vi "Dashboard Main.vi"() -> ()   [LabVIEW 2017]
uses:
  <vilib>/Rock Robotics/WPI/ThirdParty/Sensors/navX/_TypeDefs/FRIC_navX_DeviceNumbersTypeDef.ctl
  <vilib>/Utility/miscctls.llb/LVRowAndColumnTypeDef.ctl
  <vilib>/event_ctls.llb/eventvkey.ctl
  <vilib>/Rock Robotics/Network Tables/NT Read Numeric Array.vi
  <vilib>/Rock Robotics/Network Tables/NT Write Boolean.vi
  <vilib>/Rock Robotics/Network Tables/NT Read Raw.vi
  <vilib>/Rock Robotics/Network Tables/NT Write Variant.vi
  <vilib>/Rock Robotics/Network Tables/NT Read Boolean.vi
  <vilib>/Rock Robotics/WPI/Dashboard/WPI_DashboardLogging Global.vi
panel:
  in  "On/Off  2":bool caption="Solenoid"
  in  "On/Off  2":bool caption="Solenoid"
  in  "Camera Settings Right":T1={"Frame Rate"=30, "Compression"=30, "Size"=1, "DB Camera Config"=FALSE} {"Frame Rate" scale=1.0..30.0; "Compression" scale=100.0..-1.0; "Size" items=["640x480", "320x240", "160x120"]}
  in  "Camera Name Right":string(combo)="No Camera Selection"
  out "Camera Info":cluster{"Mbps LED":bool, "Mbps":dbl, "fps":dbl} {"fps" format="%#.1g"; "Mbps" format="%#.1g"}
  in  "Camera Settings":T1={"Frame Rate"=30, "Compression"=30, "Size"=1, "DB Camera Config"=FALSE} {"Frame Rate" scale=1.0..30.0; "Compression" scale=100.0..-1.0; "Size" items=["640x480", "320x240", "160x120"]}
  in  "TCP":refnum<k5>
  in  "Rec Mode":enum32{"Stop", "Record", "Playback"}(radio)
  out "Robot IP":string
  out "Image Message":string="Timeout in Camera Communications"
  in  "Dashboard Tab":T2(tab)
  in  "DancePad?":bool
  out "Reverse":bool
  in  "Auto Wait":dbl
  in  "Start Positions":string(combo)="Select Autonomous ..."
  out "NT Connection":bool
  out "MotorChart R":cluster{"Numeric":dbl, "Numeric":dbl}(graph)
  out "MotorChart L":cluster{"Numeric":dbl, "Numeric":dbl}(graph)
  out "MotorSliders R":cluster{"MotorSlide1":dbl, "MotorSlide2":dbl} {"MotorSlide2" scale=-1.0..1.0 scale format="%#_2e"; "MotorSlide1" scale=-1.0..1.0 scale format="%#_2e"}
  out "MotorSliders L":cluster{"MotorSlide1":dbl, "MotorSlide2":dbl} {"MotorSlide2" scale=-1.0..1.0 scale format="%#_2e"; "MotorSlide1" scale=-1.0..1.0 scale format="%#_2e"}
  out "Gyro":dbl(knob) scale=-180.0..180.0
  out "JS1 Z":dbl(slide) scale=-1.0..1.0 scale format="%#_2e"
  out "JS1 Graph":cluster{"X":dbl, "Y":dbl}[](graph)
  out "JS1 Buttons":T3
  out "JS2 Z":dbl(slide) scale=-1.0..1.0 scale format="%#_2e"
  out "JS2 Graph":cluster{"X":dbl, "Y":dbl}[](graph)
  out "JS2 Buttons":T3
  out "Mode":T4(ring)=enum."Auto Disabled"
  in  "Auton Goalos":string(combo)="Select Autonomous ..."
  out "Slow":bool
  out "Linear Acceleration":T5
  in  "Zero":bool
  out "Camera Image Right":T6(plugin-control)
  in  "DB/String 9":string
  in  "DB/String 8":string
  in  "DB/String 7":string
  in  "DB/String 6":string
  in  "DB/String 5":string
  in  "DB/String 4":string
  in  "DB/String 3":string
  in  "DB/String 2":string
  in  "DB/String 1":string
  in  "DB/String 0":string
  in  "DB/Slider 0":dbl(slide) scale=0.0..5.0
  in  "DB/Slider 1":dbl(slide) scale=0.0..5.0
  in  "DB/Slider 2":dbl(slide) scale=0.0..5.0
  in  "DB/Slider 3":dbl(slide) scale=0.0..5.0
  out "DB/LED 3":bool
  out "DB/LED 2":bool
  out "DB/LED 1":bool
  out "DB/LED 0":bool
  in  "DB/Button 3":bool
  in  "DB/Button 2":bool
  in  "DB/Button 1":bool
  in  "DB/Button 0":bool caption="New Name"
  in  "Use Test PWMs\n(leave off for robot":bool
  in  "Auton Game Data Override for Testing":T7
  out "Vision Values":T8
  in  "Test Slider":dbl(slide) scale=0.0..100.0 scale format="%#_3g"
  in  "On/Off":bool caption="Solenoid"
  in  "Test Name":u16(ring) items=["Select the test to run..."]
  in  "Test Tree":string(tree)
  in  "Motor":cluster{"Value":dbl, "Enable":bool} {"Value" scale=-1.0..1.0 scale format="%#_3g"}
  out "Progress":T9 {"Test Progress" scale=0.0..100.0}
  in  "Rev/Fwd":cluster{"Forward":bool, "Reverse":bool}
  in  "Test Ring":u16(ring) items=["Monochrome", "Color"]
  out "Cmd Status":string
  in  "Execute Command":bool
  in  "Command Params":string[][](table)
  in  "Command Selection":i32(listbox)
  in  "CheckList":i32(listbox)
  out "Tree":string(tree)
  out "Camera Image":T6(plugin-control)
  in  "Camera Name":string(combo)="No Camera Selection"
  # "HW"
  # "HW"
  # "Joysticks"
  # "Drive Motors"
  # "Front"
  # "Right"
  # "Left"
  # "Back"
  # "This tab is a great place for autonomous settings and robot-specific values.\nPlace controls and indicators inside this tab and match name to\nDashboard Variables on robot. You can also delete this comment."
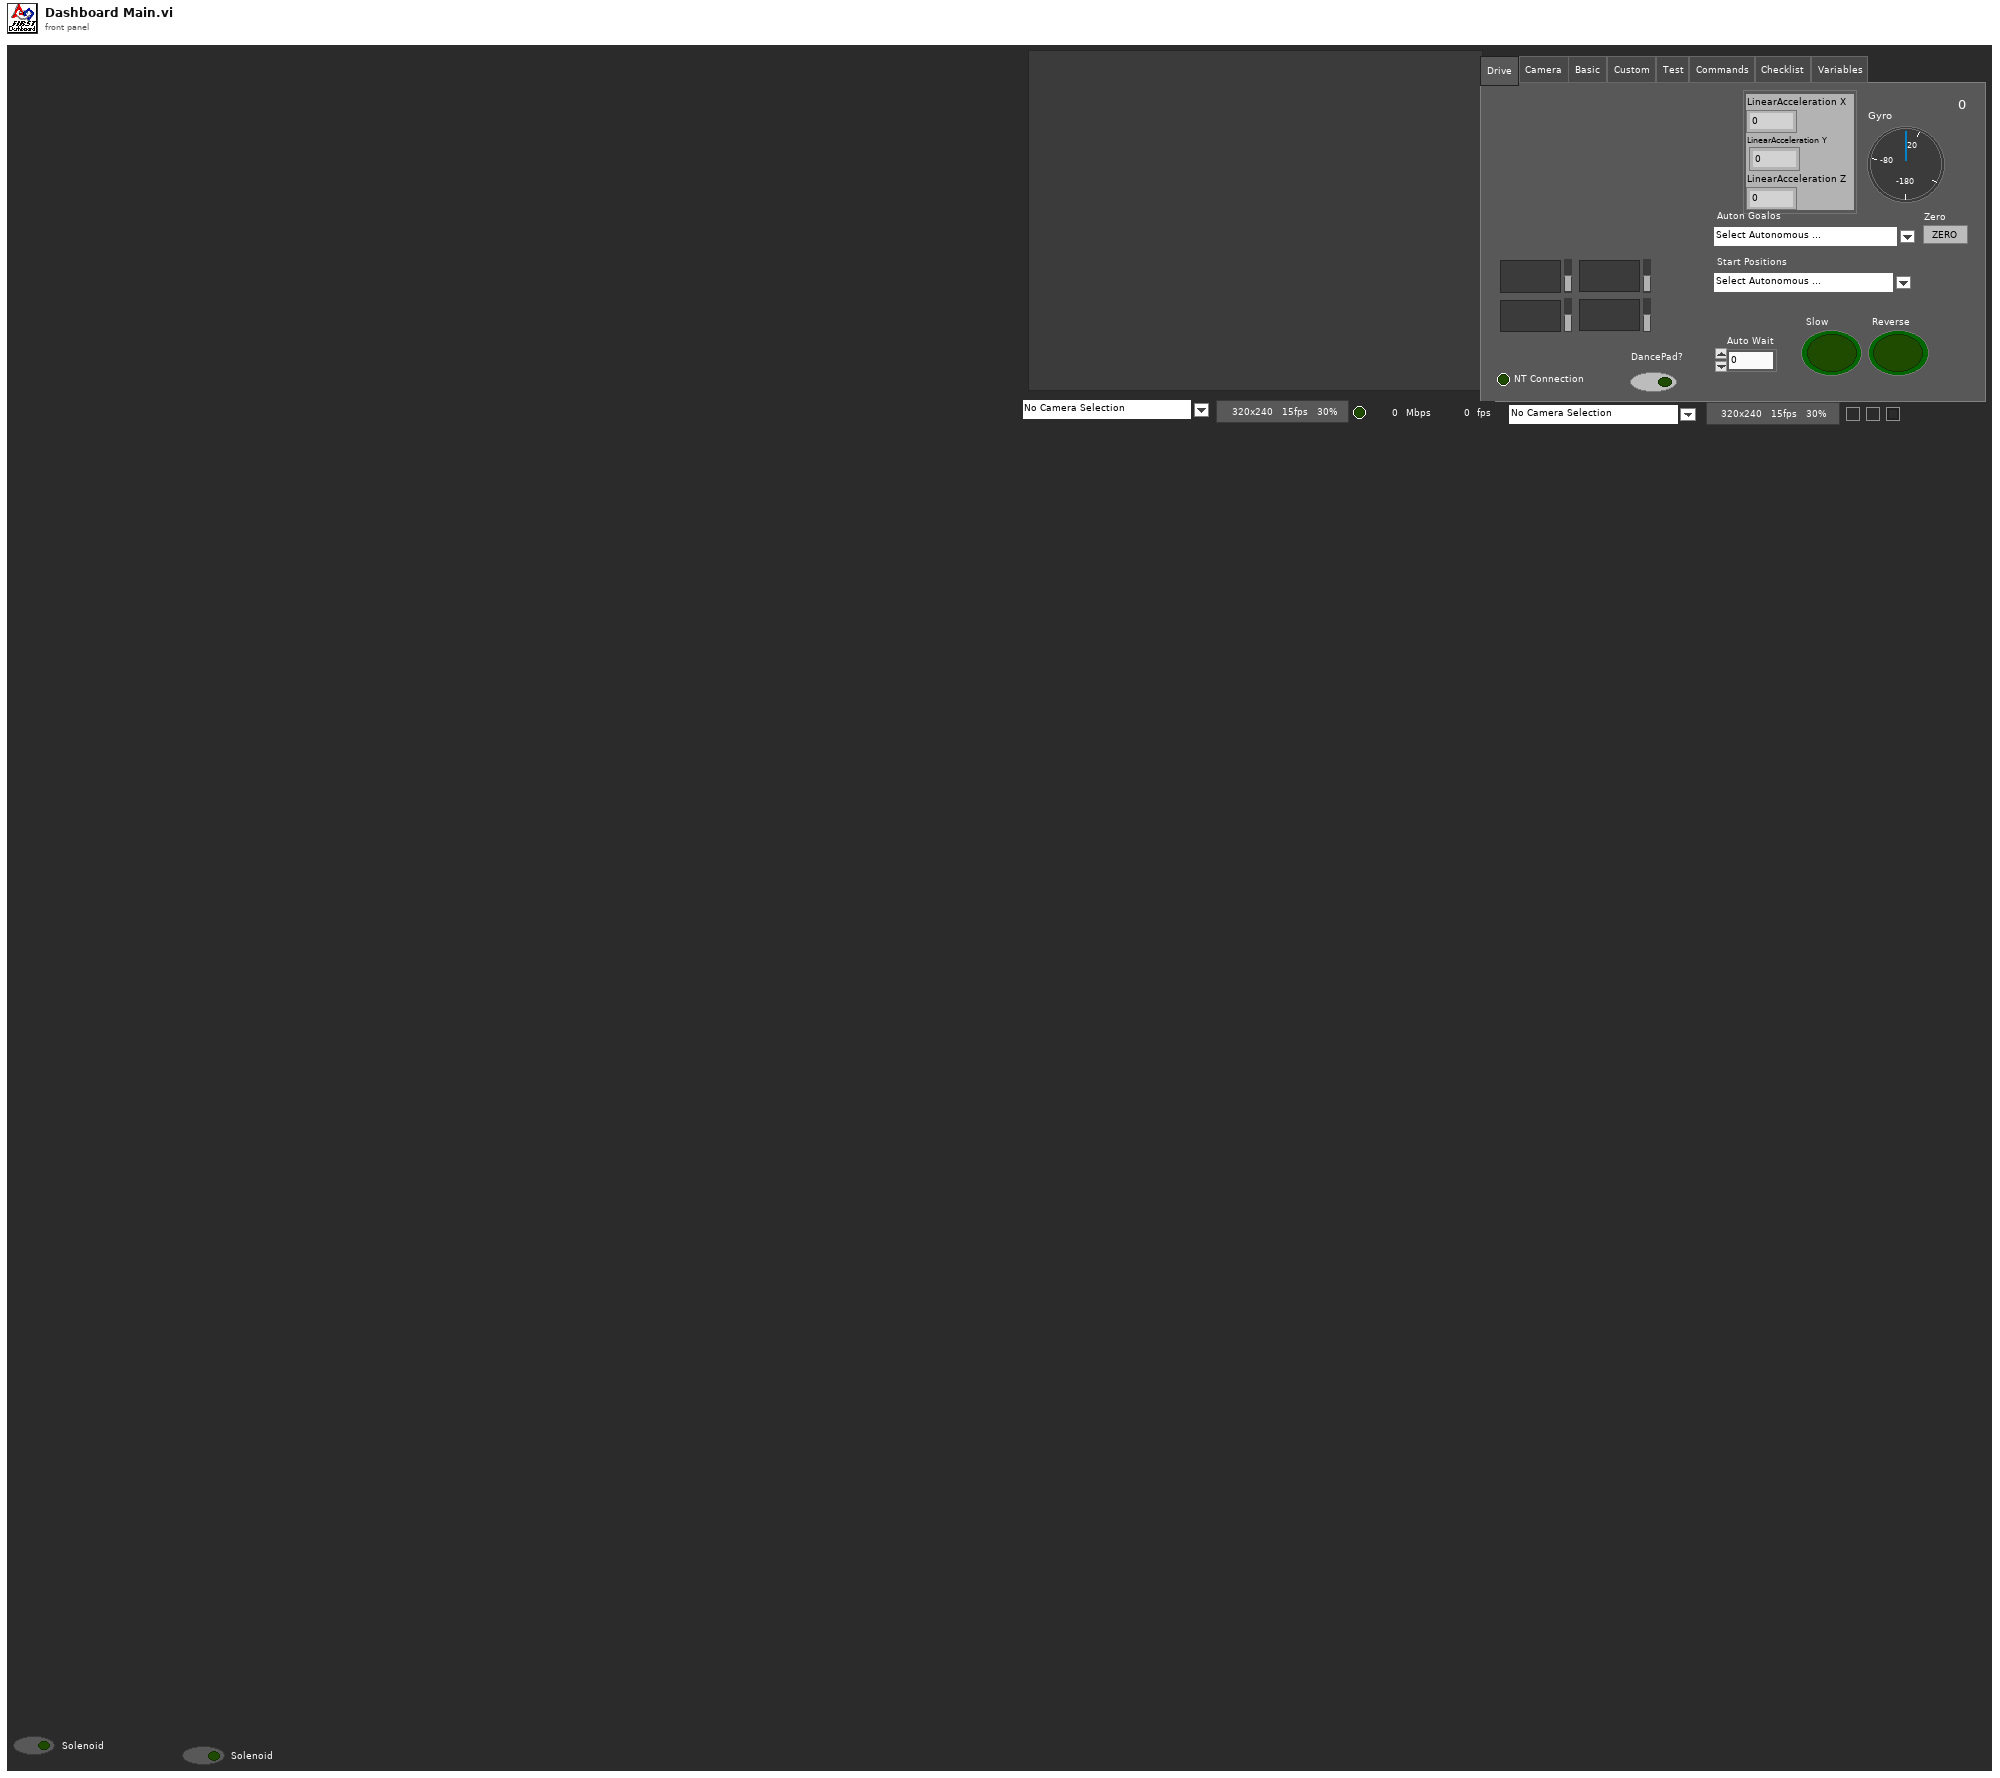
[diagram p1: front panel]
types:
  T1 = cluster{"Frame Rate":i32, "Compression":i32, "Size":u16, "DB Camera Config":bool}
  T2 = enum32{"Drive", "Camera", "Basic", "Custom", "Test", "Commands", "Checklist", "Variables"}
  T3 = cluster{bool, bool, bool, bool, bool, bool, bool, bool, bool, bool, bool, bool}
  T4 = enum8{"Tele-Op Disabled", "Tele-Op Enabled", "Auto Disabled", "Auto Enabled", "Test Disabled", "Test Enabled", "Disconnected", "No Code", "E-Stop"}
  T5 = cluster{"LinearAcceleration X":dbl, "LinearAcceleration Y":dbl, "LinearAcceleration Z":dbl}
  T6 = typedef "IMAQ Image.ctl" = refnum<image>
  T7 = cluster{"Enable":bool, "Switch Left":bool, "Scale Left":bool}
  T8 = cluster{"Center of Mass X":dbl, "Turn degrees":dbl, "Pixel Area":dbl, "Positive or Negative?":dbl}
  T9 = cluster{"Test Progress":u8, "Test Progress Text":string}
  T10 = typedef "FRIC_navX_DeviceNumbersTypeDef.ctl" = enum16{"Dev0", "Dev1", "Dev2", "Dev3"}
  T11 = cluster{"Save Path":path, "Interval (s)":dbl, "Keep":i32}
  T12 = typedef "Image Type" = u32
  T13 = cluster{"IDs":cluster{"RPC field ID":u16, "Unique ID":u16}, "String":string}
  T14 = cluster{"Error Strings":string, "Disable Counts":cluster{u16, u16}, "Rail Faults":cluster{u16, u16, u16}, "Robot IP":string, "DB Mode":u8, "Event Info":cluster{"Name":string, "Type":u8, "Number":u16, "Replay":u8}}
  T15 = cluster{"Storage":cluster{"Disk Free":u64, "RAM Block":u32, "RAM free":u32}, "CPU Utilization":cluster{"CPU % ISR":sgl, "CPU % Time Crit":sgl, "CPU % Timed Str":sgl, "CPU % High":sgl, "CPU % Above":sgl, "CPU % Normal":sgl, "CPU % Low":sgl}, "CAN":cluster{"% Bus Utilization":sgl, "Bus Off Cnt":u32, "TX_FIFO Full Cnt":u32, "Receive Error Cnt":u8, "Transmit Error Cnt":u8}, "HID":cluster{"HID Outputs":u32, "Rumble Low":u16, "Rumble High":u16}[]}
  T16 = cluster{"Status bits":cluster{"Test Mode":bool, "Autonomous":bool, "Enabled":bool, "Code Start":bool, "Brownout":bool, "Reserved 2":bool, "Reserved 3":bool, "E-Stop":bool}, "Code Trace":cluster{"Disabled":bool, "TeleOp":bool, "Auto":bool, "Test":bool}, "Controller Type":enum16{"unknown", "cRIO", "roboRio"}, "Code?":enum16{"unknown", "noCode", "code"}, "Battery V":dbl}
  T17 = cluster{"Control Bits":cluster{"TestMode":bool, "Autonomous":bool, "Enabled":bool, "FMS Present":bool, bool, bool, bool, "E-Stop":bool}, "Team Station ":u8, "Countdown":sgl, "Joystick Values":cluster{"Axes":dbl[], "Buttons":bool[], "POVs":i16[]}[]}
  T18 = cluster{"Axes":dbl[], "Buttons":bool[], "POVs":i16[]}[]
  T19 = cluster{"Axes":dbl[], "Buttons":bool[], "POVs":i16[]}
  T20 = cluster{"Buttons[0]":bool, "Buttons[1]":bool, "Buttons[2]":bool, "Buttons[3]":bool, "Buttons[4]":bool, "Buttons[5]":bool, "Buttons[6]":bool, "Buttons[7]":bool, "Buttons[8]":bool, "Buttons[9]":bool, "Buttons[10]":bool, "Buttons[11]":bool}
  T21 = cluster{"Camera Image":refnum<vi>, "Dashboard Tab":refnum<vi>, "On/Off ":refnum<vi>, "Rec Mode":refnum<vi>, "Test Slider":refnum<vi>, "On/Off ":refnum<vi>, "Test Ring":refnum<vi>, "Rev/Fwd":refnum<vi>, "Test Name":refnum<vi>, "Motor":refnum<vi>, "Progress":refnum<vi>, "CheckList":refnum<vi>, "Tree":refnum<vi>, "Test Tree":refnum<vi>, "Command Params":refnum<vi>, "Command Selection":refnum<vi>, "Execute Command":refnum<vi>, "Cmd Status":refnum<vi>, "Camera Settings":refnum<vi>, "Camera Name":refnum<vi>, "Camera Info":refnum<vi>, "Camera Settings Right":refnum<vi>, "Camera Name Right":refnum<vi>, "Camera Image Right":refnum<vi>}
  T22 = cluster{"Camera Name":string, string, "Saved DB Images Info":cluster{"Save Path":path, "Interval (s)":dbl, "Keep":i32}}
  T23 = cluster{"Camera Name Right":string, string, "Saved DB Images Info":cluster{"Save Path":path, "Interval (s)":dbl, "Keep":i32}}
  T24 = cluster{"Operation":enum16{"Update", "Clear"}, "Color Box":u32}[]
  T25 = typedef "eventvkey.ctl" = enum16{"ASCII", "Enter", "Return", "Shift", "Ctrl", "Alt", "Cmd", "Opt", "Caps", "NumLock", "Clear", "Break", "Up", "Down", "Left", "Right", "Insert", "Delete", "Home", "End", "PageUp", "PageDown", "Escape", "Help", "Pause", "ScrollLock", "F1", "F2", "F3", "F4", "F5", "F6", "F7", "F8", "F9", "F10", "F11", "F12", "F13", "F14", "F15", "F16", "F17", "F18", "F19", "F20", "F21", "F22", "F23", "F24", "Play", "VolumeUp", "VolumeDown", "Mute", "Two Byte Char"}
  T26 = cluster{"Image Size":bool, "Image Type":bool, "Pixel Value":bool, "ROI Information":bool, "Zoom Factor":bool}
  T27 = cluster{"Operation":enum16{"Update", "Clear"}, "Color Box":u32}
  T28 = typedef "LVRowAndColumnTypeDef.ctl" = cluster{"Row":i32, "Column":i32}
  T29 = cluster{"Shift":bool, "Ctrl":bool, "Alt":bool, "Cmd":bool, "Opt":bool}
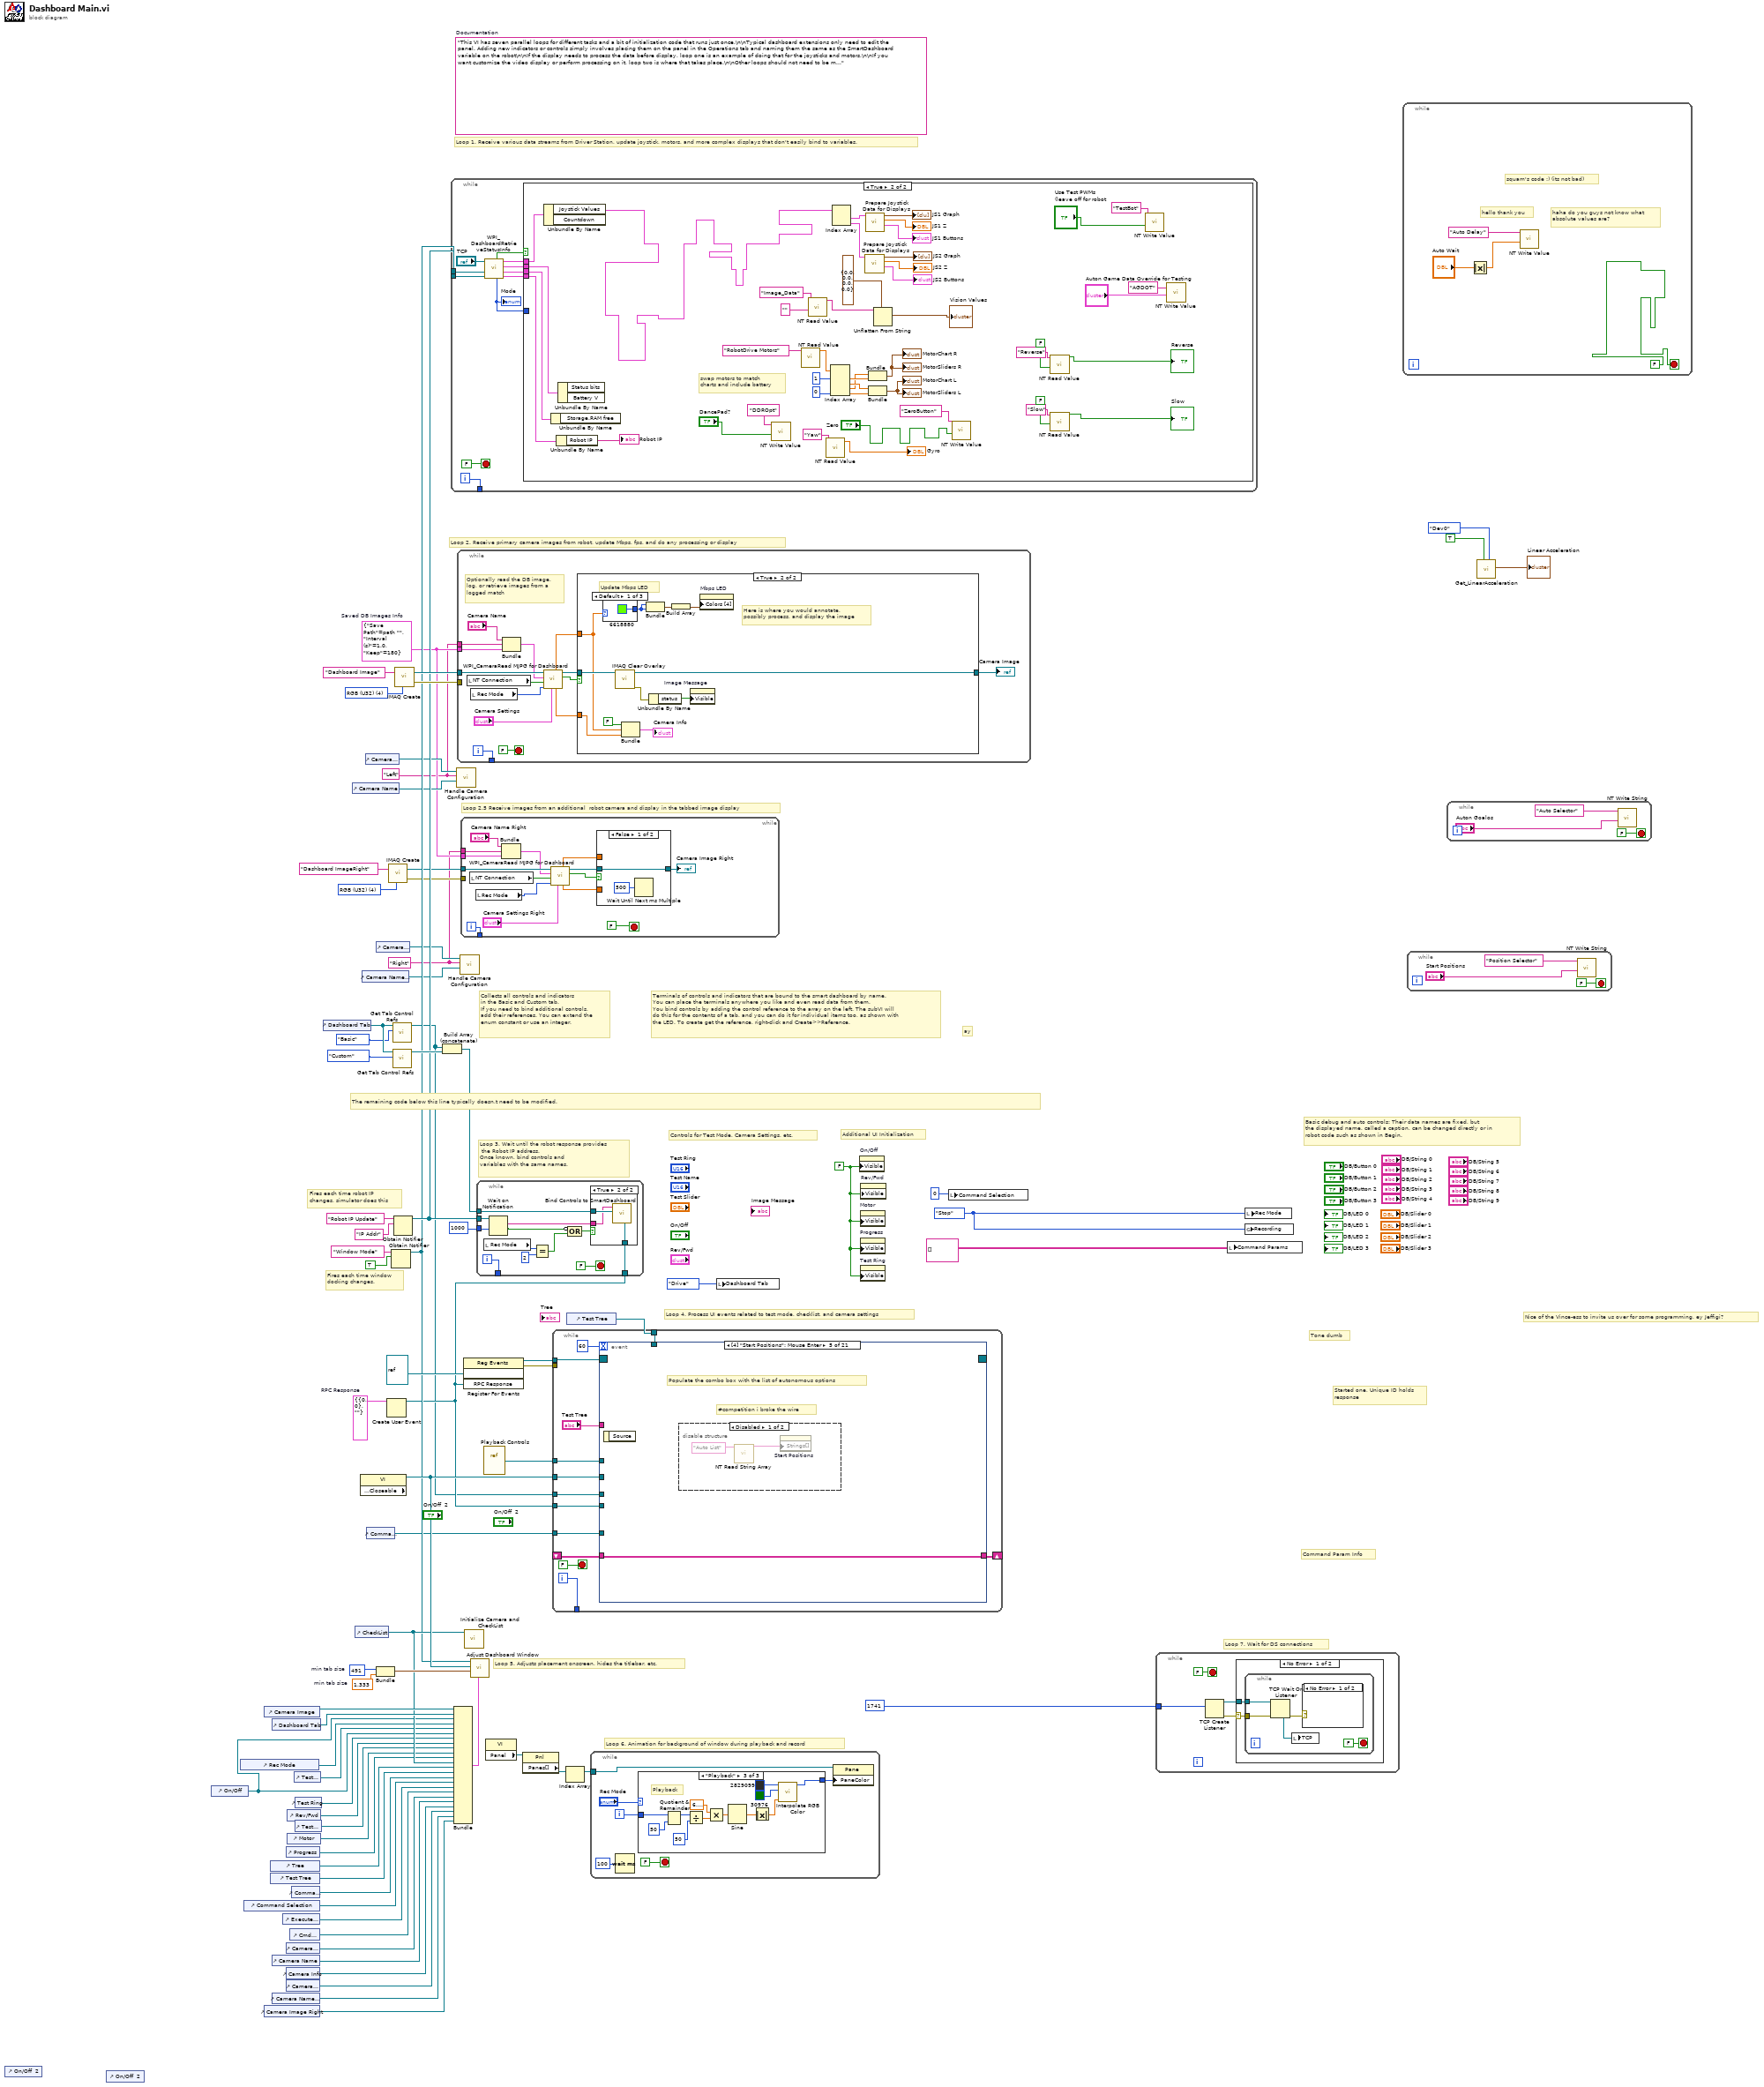
[diagram p0: block diagram]
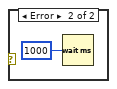
[diagram p3: hidden frame]
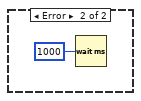
[diagram p4: hidden frame]
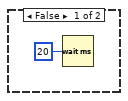
[diagram p5: hidden frame]
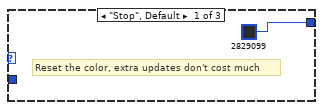
[diagram p6: hidden frame]
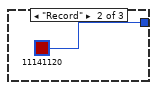
[diagram p7: hidden frame]
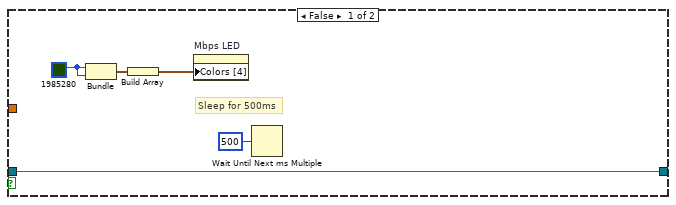
[diagram p9: hidden frame]
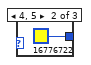
[diagram p10: hidden frame]
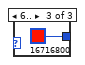
[diagram p11: hidden frame]
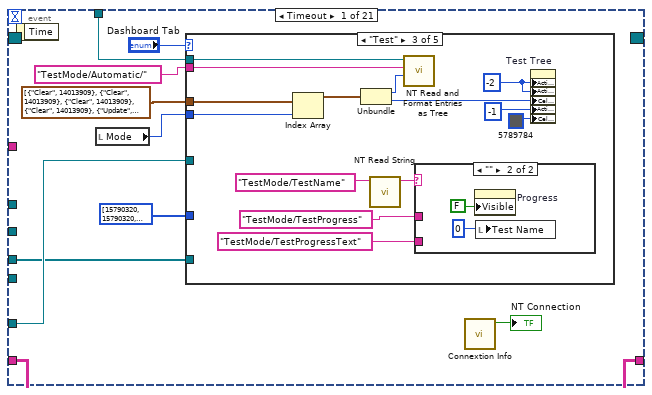
[diagram p12: hidden frame]
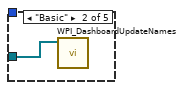
[diagram p14: hidden frame]
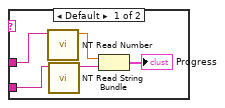
[diagram p15: hidden frame]
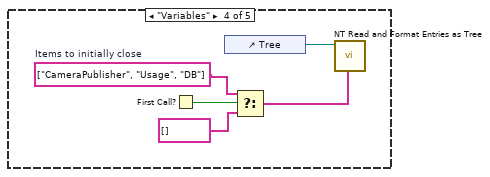
[diagram p16: hidden frame]
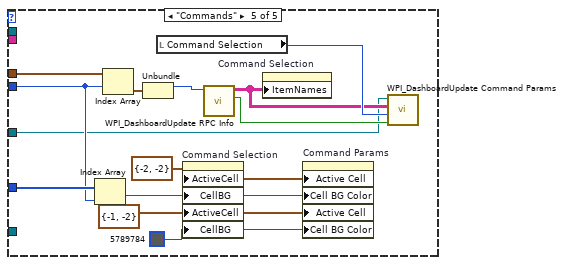
[diagram p17: hidden frame]
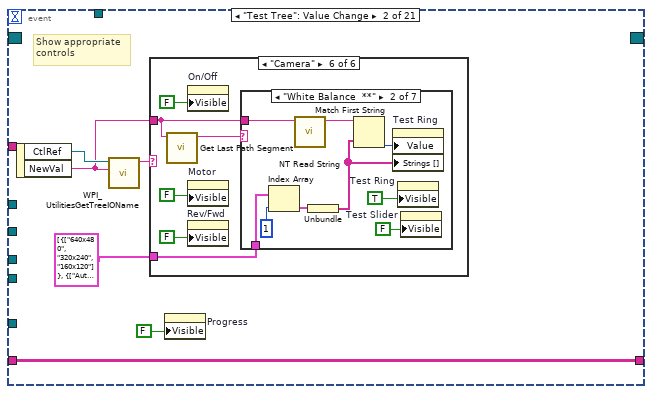
[diagram p18: hidden frame]
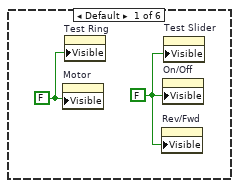
[diagram p19: hidden frame]
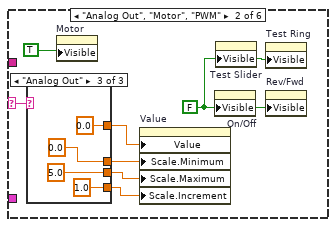
[diagram p20: hidden frame]
diagram:
  w7 = T11 {"Save Path"=path "", "Interval (s)"=1.0, "Keep"=180}  # Saved DB Images Info
  w6 = "Right"
  w5 = "Left"
  w17 = T12 4 items=["Grayscale (U8)", "Grayscale (I16)", "Grayscale (SGL)", "Complex (CSG)", "RGB (U32)", "HSL (U32)", "RGB (U64)"] ("Image Type")
  w31 = T13 {"IDs"={"RPC field ID"=0, "Unique ID"=0}, "String"=""}  # RPC Response
  w52 = 491  # min tab size
  w51 = 1.333  # min tab size
  w59 = enum32{"Stop", "Record", "Playback"}."Stop" ("Rec Mode")
  w38 = FALSE ("Visible")
  (unwired) "This VI has seven parallel loops for different tasks and a bit of initialization code that runs just once.\n\nTypical dashboard extensions only need to edit the panel. Adding new indicators or controls simply involves placing them on the panel in the Operations tab and naming them the same as the SmartDashboard variable on the robot\n\nIf the display needs to process the data before display, loop one is an example of doing that for the joysticks and motors.\n\nIf you want customize the video display or perform processing on it, loop two is where that takes place.\n\nOther loops should not need to be modified. They are pretty standard, and document the task they perform."  # Documentation
  w76 = T12 4 items=["Grayscale (U8)", "Grayscale (I16)", "Grayscale (SGL)", "Complex (CSG)", "RGB (U32)", "HSL (U32)", "RGB (U64)"] ("Image Type")
  # "ay"
  # "Nice of the Vince-ess to invite us over for some programming, ey Jeffigi?"
  # "Tone dumb"
  # "Loop 2.5 Receive images from an additional  robot camera and display in the tabbed image display"
  # "Command Param Info"
  # "Started one, Unique ID holds\nresponse"
  # "Loop 7. Wait for DS connections"
  # "Basic debug and auto controls: Their data names are fixed, but\nthe displayed name, called a caption, can be changed directly or in\nrobot code such as shown in Begin."
  # "Controls for Test Mode, Camera Settings, etc."
  # "Additional UI Initialization"
  # "Loop 6. Animation for background of window during playback and record"
  # "Fires each time robot IP\nchanges, simulator does this"
  # "Fires each time window\ndocking changes."
  # "Collects all controls and indicators\nin the Basic and Custom tab.\nIf you need to bind additional controls,\nadd their references. You can extend the\nenum constant or use an integer."
  # "The remaining code below this line typically doesn,t need to be modified."
  # "Loop 4. Process UI events related to test mode, checklist, and camera settings"
  # "Terminals of controls and indicators that are bound to the smart dashboard by name.\nYou can place the terminals anywhere you like and even read data from them.\nYou bind controls by adding the control reference to the array on the left. The subVI will\ndo this for the contents of a tab, and you can do it for individual items too, as shown with\nthe LED. To create get the reference, right-click and Create>>Reference."
  # "Loop 3. Wait until the robot response provides\n the Robot IP address.\nOnce known, bind controls and\nvariables with the same names."
  # "Loop 5. Adjusts placement onscreen, hides the titlebar, etc."
  # "Loop 1. Receive various data streams from Driver Station, update joystick, motors, and more complex displays that don't easily bind to variables."
  # "Loop 2. Receive primary camera images from robot, update Mbps, fps, and do any processing or display"
  n1 = control-ref of="On/Off  2"() -> ()  [unwired: 1 out]
  n2 = control-ref of="On/Off  2"() -> ()  [unwired: 1 out]
  n3 = control-ref of="On/Off"() -> (w4:refnum<vi>)
  n4 = control-ref of="Rec Mode"() -> (w43:refnum<vi>)
  n5 = control-ref of="Command Selection"() -> (w30:refnum<vi>)
  n6 = control-ref of="Camera Image Right"() -> (w10:refnum<vi>)
  n7 = control-ref of="Camera Image"() -> (w54:refnum<vi>)
  n8 = control-ref of="Tree"() -> (w47:refnum<vi>)
  n9 = control-ref of="Test Tree"() -> (w46:refnum<vi>)
  n10 = control-ref of="Dashboard Tab"() -> (w53:refnum<vi>)
  n11 = control-ref of="Camera Name"() -> (w21:refnum<vi>)
  n12 = control-ref of="Camera Name Right"() -> (w11:refnum<vi>)
  n13 = control-ref of="Execute Command"() -> (w32:refnum<vi>)
  n14 = control-ref of="Progress"() -> (w39:refnum<vi>)
  n15 = control-ref of="Camera Settings"() -> (w22:refnum<vi>)
  n16 = control-ref of="Camera Info"() -> (w20:refnum<vi>)
  n17 = control-ref of="Camera Settings Right"() -> (w12:refnum<vi>)
  n18 = control-ref of="Rev/Fwd"() -> (w40:refnum<vi>)
  n19 = control-ref of="Motor"() -> (w44:refnum<vi>)
  n20 = control-ref of="Cmd Status"() -> (w26:refnum<vi>)
  n21 = control-ref of="Command Params"() -> (w33:refnum<vi>)
  n22 = control-ref of="Test Slider"() -> (w42:refnum<vi>)
  n23 = control-ref of="Test Ring"() -> (w41:refnum<vi>)
  n24 = control-ref of="Test Name"() -> (w45:refnum<vi>)
  n25 = control-ref of="Dashboard Tab"() -> (w57:refnum<vi>)
  n26 = control-ref of="Camera Name"() -> (w23:refnum<vi>)
  n27 = control-ref of="CheckList"() -> (w48:refnum<vi>)
  n28 = property class="VI" props=["Front Panel.Closeable"]() -> (reference out=w58:refnum<vi>)  [unwired: 2 in, 2 out]
  n29 = control-ref of="Camera Name Right"() -> (w13:refnum<vi>)
  n30 = control-ref of="Camera Settings"() -> (w24:refnum<vi>)
  n31 = control-ref of="Command Params"() -> (w25:refnum<vi>)
  n32 = control-ref of="Camera Settings Right"() -> (w14:refnum<vi>)
  n33 = Bundle("min tab size"=w52, "min tab size"=w51) -> (w50:cluster{"min tab size":i32, "min tab size":dbl})  [unwired: 1 in]
  n34 = Create User Event(user event datatype=w31) -> (user event=w27:refnum<user-event>)  [unwired: 1 in, 1 out]
  n35 = call "IMAQ Create"("Image Name"="Dashboard ImageRight", "Image Type"=w17) -> ("New Image"=w16:T6, "error out"=w15:errorcluster)  [unwired: 2 in, 1 out]
  n36 = Obtain Notifier(name (unnamed)="Window Mode", notification data type=TRUE) -> (notifier out=w36:refnum<notifier>)  [unwired: 2 in, 2 out]
  n37 = call <vilib>:"Get Tab Control Refs.vi"("Page Index"=T2."Basic" ("Dashboard Tab"), "TabControl in"=w57) -> ("ControlsOnPage"=w19:refnum<vi>[])  [unwired: 9 in]
  n38 = call <vilib>:"Get Tab Control Refs.vi"("Page Index"=T2."Custom" ("Dashboard Tab"), "TabControl in"=w57) -> ("ControlsOnPage"=w56:refnum<vi>[])  [unwired: 9 in]
  n39 = Obtain Notifier(name (unnamed)="Robot IP Update", notification data type="IP Addr" ("name (unnamed)")) -> (notifier out=w37:refnum<notifier>)  [unwired: 2 in, 2 out]
  n40 = call "IMAQ Create"("Image Name"="Dashboard Image", "Image Type"=w76) -> ("New Image"=w74:T6, "error out"=w73:errorcluster)  [unwired: 2 in, 1 out]
  n41 = Build Array (concatenate)(w19, w56) -> (w55:refnum<vi>[])
  n42 = while {
    tunnel: [w86] -> _
    tunnel: w37 -> [w80]
    tunnel: w36 -> [w77]
    i -> [w86]
    stop <- FALSE stop-if-true
    n43 = call <vilib>:"WPI_DashboardRetrieveStatusInfo.vi"("Binding Refnum"=w80, "Window Mode Notifier"=w77, "TCP Cnx"="TCP") -> ("Power and Errors"=w81:T14, "Robot Metrics"=w84:T15, "Status Info"=w85:T16, "Control Info"=w82:T17, "Robot Mode"=w79:T4, "Process?"=w83:bool)  [unwired: 3 in]
    "Mode" <- w79
    n44 = case shown="True" w83 {
      tunnel: w85 -> [_ w133]
      tunnel: w84 -> [_ w132]
      tunnel: w82 -> [_ w131]
      tunnel: w81 -> [_ w130]
      tunnel: w79 -> [_ _]
      frame False {
        n45 = Wait (ms)(milliseconds to wait=u32 20) -> ()  [unwired: 1 out]
      }
      frame True {
        # "swap motors to match\ncharts and include battery"
        n46 = Unbundle By Name(w131) -> ("Joystick Values"=w89:T18)  [unwired: 1 out]
        n47 = Unbundle By Name(w132) -> ()  [unwired: 1 out]
        n48 = Unbundle By Name(w130) -> ("Robot IP"=→"Robot IP":string)
        n49 = Unbundle By Name(w133) -> ()  [unwired: 2 out]
        n50 = call-poly <vilib>:"NT Write Value.vi"("Boolean"="DancePad?", "Name"="DDROpt") -> ()  [unwired: 9 in, 1 out]
        n51 = call-poly <vilib>:"NT Read Value.vi"("Name"="RobotDrive Motors") -> ("Numeric Array"=w112:dbl[])  [unwired: 9 in, 1 out]
        n52 = call-poly <vilib>:"NT Read Value.vi"("Default Value"="", "Name"="Image_Data") -> ("Raw"=w105:string)  [unwired: 8 in, 1 out]
        n53 = call-poly <vilib>:"NT Read Value.vi"("Name"="Yaw") -> ("Numeric"=→"Gyro":dbl)  [unwired: 9 in, 1 out]
        n54 = Index Array(array=w112, index #1=1, index #4=0) -> (element #1=w125:dbl, element #2=w126:dbl, element #3=w124:dbl, element #4=w129:dbl)  [unwired: 2 in]
        n55 = Index Array(array=w89) -> (element #1=w121:T19, element #2=w117:T19)  [unwired: 2 in]
        n56 = call "Prepare Joystick Data for Displays.vi"("Joystick Values"=w117) -> ("Buttons"=→"JS2 Buttons":T20, "Z Axis"=→"JS2 Z":dbl, "Cartesian Data"=→"JS2 Graph":cluster{"X axis":dbl, "X axis":dbl}[])  [unwired: 8 in]
        n57 = call "Prepare Joystick Data for Displays.vi"("Joystick Values"=w121) -> ("Buttons"=→"JS1 Buttons":T20, "Z Axis"=→"JS1 Z":dbl, "Cartesian Data"=→"JS1 Graph":cluster{"X axis":dbl, "X axis":dbl}[])  [unwired: 8 in]
        n58 = Bundle("Numeric"=w124, "Numeric"=w125) -> (→"MotorChart R" →"MotorSliders R":cluster{"Numeric":dbl, "Numeric":dbl})  [unwired: 1 in]
        n59 = Bundle("Numeric"=w126, "Numeric"=w129) -> (→"MotorChart L" →"MotorSliders L":cluster{"Numeric":dbl, "Numeric":dbl})  [unwired: 1 in]
        n60 = Unflatten From String(type=T8 {"Center of Mass X"=0.0, "Turn degrees"=0.0, "Pixel Area"=0.0, "Positive or Negative?"=0.0} ("Cluster"), binary string=w105) -> (value=→"Vision Values":T8)  [unwired: 3 in, 2 out]
        n61 = call-poly <vilib>:"NT Write Value.vi"("Boolean"="Zero", "Name"="ZeroButton") -> ()  [unwired: 9 in, 1 out]
        n62 = call-poly <vilib>:"NT Read Value.vi"("Default Value"=FALSE, "Name"="Reverse") -> ("Boolean"=→"Reverse":bool)  [unwired: 8 in, 1 out]
        n63 = call-poly <vilib>:"NT Read Value.vi"("Default Value"=FALSE, "Name"="Slow") -> ("Boolean"=→"Slow":bool)  [unwired: 8 in, 1 out]
        n64 = call-poly <vilib>:"NT Write Value.vi"("Boolean"="Use Test PWMs\n(leave off for robot", "Name"="TestBot") -> ()  [unwired: 9 in, 1 out]
        n65 = call-poly <vilib>:"NT Write Value.vi"("Variant"="Auton Game Data Override for Testing", "Name"="AGDOT") -> ()  [unwired: 9 in, 1 out]
      }
    }
  }
  n66 = Bundle("Camera Image"=w54, "Dashboard Tab"=w53, "On/Off"=w4, "Rec Mode"=w43, "Test Slider"=w42, "On/Off"=w4, "Test Ring"=w41, "Rev/Fwd"=w40, "Test Name"=w45, "Motor"=w44, "Progress"=w39, "CheckList"=w48, "Tree"=w47, "Test Tree"=w46, "Command Params"=w33, "Command Selection"=w30, "Execute Command"=w32, "Cmd Status"=w26, "Camera Settings"=w22, "Camera Name"=w21, "Camera Info"=w20, "Camera Settings Right"=w12, "Camera Name Right"=w11, "Camera Image Right"=w10) -> (w49:T21)  [unwired: 1 in]
  n67 = call "Handle Camera Configuration.vi"("CameraNameRef"=w23, "Display Name"=w5, "ClusterRef"=w24) -> ()  [unwired: 9 in]
  n68 = while {
    tunnel: w74 -> [w146]
    tunnel: w73 -> [_]
    tunnel: [w147] -> _
    tunnel: w7 -> [w137]
    tunnel: w5 -> [w134]
    i -> [w147]
    stop <- FALSE stop-if-true
    # "Optionally read the DB image,\nlog, or retrieve images from a\nlogged match"
    n69 = local read "NT Connection"() -> (w138:bool)
    n70 = local read "Rec Mode"() -> (w142:enum32{"Stop", "Record", "Playback"})
    n71 = Bundle("Camera Name"="Camera Name", w134, "Saved DB Images Info"=w137) -> (w136:T22)  [unwired: 1 in]
    n72 = call <vilib>:"WPI_CameraRead MJPG for Dashboard.vi"("Camera Settings"="Camera Settings", "Rec Mode"=w142, "NT Connection"=w138, "Capture Info"=w136, "Refnum in"=w146) -> ("Active"=w144:bool, "Refnum out"=w145:T6, "FPS"=w143:dbl, "Bandwidth (Mbps)"=w141:dbl)  [unwired: 3 in]
    n73 = case shown="True" w144 {
      tunnel: w145 -> [w149 w160]
      tunnel: w141 -> [_ w157]
      tunnel: w143 -> [_ w158]
      tunnel: [w149 w154] -> w139
      frame False {
        w151 = u32 1985280 ("Color Box")
        # "Sleep for 500ms"
        n74 = Bundle("Color Box"=w151, "Color Box"=w151) -> (w152:cluster{"Color Box":u32, "Color Box":u32})  [unwired: 1 out]
        n75 = Build Array(w152) -> (w150:cluster{"Color Box":u32, "Color Box":u32}[])
        n76 = property on="Mbps LED" class="Bool (strict)"("Colors [4]"=w150) -> ()  [unwired: 2 in, 2 out]
        n77 = Wait Until Next ms Multiple(millisecond multiple=u32 500) -> ()  [unwired: 1 out]
      }
      frame True {
        # "Here is where you would annotate,\npossibly process, and display the image"
        # "Update Mbps LED"
        n78 = case shown="Default" w157 {
          tunnel: [u32 6618880 ("Color Box") u32 16776722 ("Color Box") u32 16716800 ("Color Box")] -> w161
          frame Default {
          }
          frame 4, 5 {
          }
          frame 6.. {
          }
        }
        n79 = call "IMAQ Clear Overlay"("Image"=w160) -> ("error out"=w163:errorcluster, "Image Out"=w154:T6)  [unwired: 2 in, 7 out]
        n80 = Bundle(FALSE, "Bandwidth (Mbps)"=w157, "FPS"=w158) -> (→"Camera Info":cluster{bool, "Bandwidth (Mbps)":dbl, "FPS":dbl})  [unwired: 1 in]
        n81 = Bundle("Color Box"=w161, "Color Box"=w161) -> (w162:cluster{"Color Box":u32, "Color Box":u32})  [unwired: 1 out]
        n82 = Unbundle By Name(w163) -> ("status"=w164:bool)
        n83 = Build Array(w162) -> (w159:cluster{"Color Box":u32, "Color Box":u32}[])
        n84 = property on="Image Message" class="Str"("Visible"=w164) -> ()  [unwired: 2 in, 2 out]
        n85 = property on="Mbps LED" class="Bool (strict)"("Colors [4]"=w159) -> ()  [unwired: 2 in, 2 out]
      }
    }
    "Camera Image" <- w139
  }
  n86 = call "Handle Camera Configuration.vi"("CameraNameRef"=w13, "Display Name"=w6, "ClusterRef"=w14) -> ()  [unwired: 9 in]
  n87 = while {
    tunnel: w16 -> [w182]
    tunnel: w15 -> [_]
    tunnel: [w177] -> _
    tunnel: w7 -> [w171]
    tunnel: w6 -> [w168]
    i -> [w177]
    stop <- FALSE stop-if-true
    n88 = local read "NT Connection"() -> (w172:bool)
    n89 = local read "Rec Mode"() -> (w181:enum32{"Stop", "Record", "Playback"})
    n90 = Bundle("Camera Name Right"="Camera Name Right", w168, "Saved DB Images Info"=w171) -> (w170:T23)  [unwired: 1 in]
    n91 = call <vilib>:"WPI_CameraRead MJPG for Dashboard.vi"("Camera Settings"="Camera Settings Right", "Rec Mode"=w181, "NT Connection"=w172, "Capture Info"=w170, "Refnum in"=w182) -> ("Active"=w176:bool, "Refnum out"=w179:T6, "FPS"=w174:dbl, "Bandwidth (Mbps)"=w175:dbl)  [unwired: 3 in]
    n92 = case shown="False" w176 {
      tunnel: w179 -> [w183 w185]
      tunnel: w175 -> [_ _]
      tunnel: w174 -> [_ _]
      tunnel: [w183 w185] -> w173
      frame False {
        n93 = Wait Until Next ms Multiple(millisecond multiple=u32 500) -> ()  [unwired: 1 out]
      }
      frame True {
      }
    }
    "Camera Image Right" <- w173
  }
  n94 = register-events(refnum<vi> refnum, w27) -> (reference out=w63:refnum<event-registration>, error out=w62:errorcluster)  [unwired: 2 in]
  n95 = call "Initialize Camera and CheckList.vi"("ListBox in"=w48) -> ()  [unwired: 11 in]
  n96 = call "Adjust Dashboard Window.vi"("Sizing Refnums"=w49, "Size Constraints"=w50, "VI"=w58, "WIn Mode"=w36) -> ()  [unwired: 8 in]
  n97 = while {
    tunnel: w55 -> [w197]
    tunnel: w37 -> [w195]
    tunnel: [w193] -> _
    tunnel: u32 1000 ("milliseconds to wait") -> [w192]
    tunnel: w27 -> [w186]
    i -> [w193]
    stop <- FALSE stop-if-true
    n98 = local read "Rec Mode"() -> (w188:enum32{"Stop", "Record", "Playback"})
    n99 = Wait on Notification(notifier=w195, timeout in ms (-1)=w192) -> (notification=w194:string, timed out?=w190:bool)  [unwired: 2 in, 2 out]
    n100 = Equal?(x=w188, y=u16 2 ("Rec Mode")) -> (x = y?=w189:bool)
    n101 = Compound Arithmetic op=OR(invert w190, w189) -> (w191:bool)
    n102 = case shown="True" w191 {
      tunnel: w197 -> [_ w200]
      tunnel: w194 -> [_ w199]
      tunnel: w186 -> [_ w198]
      frame False {
      }
      frame True {
        n103 = call <vilib>:"Bind Controls to SmartDashboard.vi"("RPC ref"=w198, "Bound Control Refs"=w200, "Server IP Address"=w199) -> ()  [unwired: 9 in]
      }
    }
  }
  n104 = vi-ref "Playback Controls.vi"() -> (w64:refnum<vi>)
  n105 = property class="VI"() -> ("Panel"=w66:refnum<vi>)  [unwired: 2 in, 2 out]
  n106 = property class="Pnl"(reference=w66) -> ("Panes[]"=w67:refnum<vi>[])  [unwired: 1 in, 2 out]
  n107 = Index Array(array=w67) -> (element=w65:refnum<vi>)  [unwired: 1 in]
  n108 = control-ref of="Test Tree"() -> (w68:refnum<vi>)
  n109 = while {
    tunnel: [w210] -> _
    tunnel: w68 -> [w209]
    tunnel: w64 -> [w208]
    tunnel: w63 -> [w207]
    tunnel: w62 -> [_]
    tunnel: w58 -> [w206]
    tunnel: w27 -> [w205]
    tunnel: w25 -> [w204]
    shift-right: [w203] -> _
    shift-left: _ -> [w202]
    tunnel: w19 -> [w201]
    i -> [w210]
    stop <- FALSE stop-if-true
    n110 = event shown="[4] \"Start Positions\": Mouse Enter" {
      selector: w207 -> [_ _ _ _ _ _ _ _ _ _ _ _ _ _ _ _ _ _ _ _ _]
      dyn-events: [_ _ _ _ _ _ _ _ _ _ _ _ _ _ _ _ w470 _ _ _ _] -> _
      timeout: u32 60 ("milliseconds to wait") -> [_ _ _ _ _ _ _ _ _ _ _ _ _ _ _ _ _ _ _ _ _]
      tunnel: w209 -> [w222 _ _ _ _ _ _ _ _ _ _ _ _ _ _ _ _ _ _ _ _]
      tunnel: "Test Tree" -> [_ _ _ _ _ _ _ _ _ _ _ w437 w445 w447 w451 w459 _ _ _ _ _]
      tunnel: w208 -> [_ _ _ _ _ _ _ _ _ _ _ _ _ _ _ _ w472 _ w490 _ _]
      tunnel: w206 -> [_ _ _ _ _ _ _ _ _ _ _ _ _ _ _ _ w468 _ _ _ _]
      tunnel: w205 -> [_ _ _ _ _ _ _ _ _ _ _ _ _ _ _ _ w466 _ _ _ _]
      tunnel: w204 -> [w217 _ _ _ _ _ w388 _ _ _ _ _ _ _ _ _ _ _ _ _ _]
      tunnel: [w216 w265 w367 w372 w380 w385 w386 w395 w405 w412 w424 w436 w443 w446 w450 w458 w465 w485 w487 w491 w504] -> w203
      tunnel: w202 -> [w216 w265 w367 w372 w380 w385 w386 _ _ w412 w424 w436 w443 w446 w450 w458 w465 w485 w487 w491 w504]
      tunnel: w201 -> [w214 _ _ _ _ _ _ _ _ _ _ _ _ _ _ _ _ _ _ _ _]
      event Timeout {
        n111 = event-data() -> ()  [unwired: 1 in, 1 out]
        n112 = local read "Mode"() -> (w219:T4)
        n113 = case shown="\"Test\"" "Dashboard Tab" {
          tunnel: w222 -> [_ _ w238 _ _]
          tunnel: "TestMode/Automatic/" ("Name Pattern") -> [_ _ w237 _ _]
          tunnel: T24 [{"Operation"=enum."Clear", "Color Box"=14013909}, {"Operation"=enum."Clear", "Color Box"=14013909}, {"Operation"=enum."Clear", "Color Box"=14013909}, {"Operation"=enum."Clear", "Color Box"=14013909}, {"Operation"=enum."Update", "Color Box"=14013909}, {"Operation"=enum."Update", "Color Box"=16777215}, {"Operation"=enum."Clear", "Color Box"=14013909}, {"Operation"=enum."Clear", "Color Box"=14013909}, {"Operation"=enum."Clear", "Color Box"=14013909}] -> [_ _ w230 _ w258]
          tunnel: w219 -> [_ _ w229 _ w257]
          tunnel: u32[] [15790320, 15790320, 15790320, 15790320, 16777215, 16777215, 15790320, 15790320, 15790320] -> [_ _ _ _ w263]
          tunnel: w217 -> [_ _ _ _ w251]
          tunnel: w214 -> [_ w224 _ _ _]
          frame "Custom", Default {
          }
          frame "Basic" {
            n114 = call <vilib>:"WPI_DashboardUpdateNames.vi"("Controls on Tab"=w224) -> ()  [unwired: 11 in]
          }
          frame "Test" {
            w236 = -2 ("Active Item:Row Number")
            n115 = Index Array(array=w230, index=w229) -> (element=w231:T27)
            n116 = Unbundle(w231) -> ("Operation"=w232:enum16{"Update", "Clear"}, "Color Box"=w233:u32)
            n117 = call <vilib>:"NT Read String.vi"("Name"="TestMode/TestName") -> ("String"=w227:string)  [unwired: 9 in, 1 out]
            n118 = call <vilib>:"NT Read and Format Entries as Tree.vi"("Operation"=w232, "Name Pattern"=w237, "Tree Refnum"=w238) -> ()  [unwired: 7 in, 2 out]
            n119 = case shown="\"\"" w227 {
              tunnel: "TestMode/TestProgress" ("Name") -> [w240 _]
              tunnel: "TestMode/TestProgressText" ("Name") -> [w239 _]
              frame Default {
                n120 = call <vilib>:"NT Read Number.vi"("Name"=w240) -> ("Numeric"=w241:dbl)  [unwired: 9 in, 1 out]
                n121 = call <vilib>:"NT Read String.vi"("Name"=w239) -> ("String"=w242:string)  [unwired: 9 in, 1 out]
                n122 = Bundle("Numeric"=w241, "String"=w242) -> (→"Progress":cluster{"Numeric":dbl, "String":string})  [unwired: 1 in]
              }
              frame "" {
                n123 = property on="Progress" class="Clust (strict)"("Visible"=FALSE) -> ()  [unwired: 2 in, 2 out]
                n124 = local write "Test Name"(u16 0) -> ()
              }
            }
            n125 = property on="Test Tree" class="Tree (strict)"("Active Item Row Number"=w236, "ActiveColNum"=w236, "CellBG"=w233, "Active Item Row Number"=-1 ("Active Item:Row Number"), "CellBG"=u32 5789784 ("Color Box")) -> ()  [unwired: 2 in, 2 out]
          }
          frame "Variables" {
            w248 = string[] ["CameraPublisher", "Usage", "DB"]  # Items to initially close
            n126 = First Call?() -> (First Call?: T/F=w249:bool)
            n127 = control-ref of="Tree"() -> (w250:refnum<vi>)
            n128 = Select(t=w248, s=w249, f=string[] []) -> (s? t:f=w246:string[])
            n129 = call <vilib>:"NT Read and Format Entries as Tree.vi"("Tags to  Close"=w246, "Tree Refnum"=w250) -> ()  [unwired: 8 in, 2 out]
          }
          frame "Commands" {
            w259 = u32 5789784 ("Color Box")
            w260 = T28 {"Row"=-1, "Column"=-2} ("Active Cell:Active Cell")
            w262 = T28 {"Row"=-2, "Column"=-2} ("Active Cell:Active Cell")
            n130 = Index Array(array=w263, index=w257) -> (element=w261:u32)
            n131 = Index Array(array=w258, index=w257) -> (element=w256:T27)
            n132 = Unbundle(w256) -> ("Operation"=w255:enum16{"Update", "Clear"})  [unwired: 1 out]
            n133 = local read "Command Selection"() -> (w254:i32)
            n134 = property on="Command Selection" class="MCListbox (strict)"("ActiveCell"=w262, "CellBG"=w261, "ActiveCell"=w260, "CellBG"=w259) -> ()  [unwired: 2 in, 2 out]
            n135 = call <vilib>:"WPI_DashboardUpdate RPC Info.vi"("Operation"=w255) -> ("update"=w253:bool, "commands"=w252:string[][])  [unwired: 9 in]
            n136 = property on="Command Selection" class="MCListbox (strict)"("ItemNames"=w252) -> ()  [unwired: 2 in, 2 out]
            n137 = property on="Command Params" class="Tbl (strict)"("Active Cell"=w262, "Cell BG Color"=w261, "Active Cell"=w260, "Cell BG Color"=w259) -> ()  [unwired: 2 in, 2 out]
            n138 = call <vilib>:"WPI_DashboardUpdate Command Params.vi"("Update"=w253, "NewVal"=w254, "Commands"=w252, "Param Tbl"=w251) -> ()  [unwired: 7 in, 1 out]
          }
        }
        n139 = call <vilib>:"Connextion Info.vi"() -> ("Connected"=→"NT Connection":bool)  [unwired: 10 in, 1 out]
      }
      event "Test Tree": Value Change {
        # "Show appropriate\ncontrols"
        n140 = event-data() -> ("CtlRef"=w268:refnum<vi>, "NewVal"=w266:string)  [unwired: 1 in]
        n141 = call <vilib>:"WPI_UtilitiesGetTreeIOName.vi"("NewVal"=w266, "TreeControl in"=w268) -> ("I/O Name"=w269:string)  [unwired: 9 in]
        n142 = case shown="\"Camera\"" w269 {
          selector: w269 -> [_ w276 _ w298 w307 _]
          tunnel: w266 -> [_ _ w295 w297 _ w314]
          tunnel: cluster{string[]}[] [{["640x480", "320x240", "160x120"]}, {["Auto", "Fixed indoor", "Fixed outdoor 1", "Fixed outdoor 2", "Fixed fluorescent 1", "Fixed fluorescent 2", "Hold current"]}, {["Auto", "Flicker-free 50 Hz", "Flicker-free 60 Hz", "Hold current"]}, {["None", "Prioritize frame rate", "Prioritize image quality"]}, {["Monochrome", "Color"]}] -> [_ _ _ _ _ w313]
          frame Default {
            w271 = FALSE ("Visible")
            w270 = FALSE ("Visible")
            n143 = property on="Motor" class="Clust (strict)"("Visible"=w270) -> ()  [unwired: 2 in, 2 out]
            n144 = property on="Test Ring" class="Ring (strict)"("Visible"=w270) -> ()  [unwired: 2 in, 2 out]
            n145 = property on="Rev/Fwd" class="Clust (strict)"("Visible"=w271) -> ()  [unwired: 2 in, 2 out]
            n146 = property on="On/Off" class="Bool (strict)"("Visible"=w271) -> ()  [unwired: 2 in, 2 out]
            n147 = property on="Test Slider" class="Slide (strict)"("Visible"=w271) -> ()  [unwired: 2 in, 2 out]
          }
          frame "Analog Out", "Motor", "PWM" {
            w277 = FALSE ("Visible")
            n148 = case shown="\"Analog Out\"" w276 {
              tunnel: [1.0 ("Value") -1.0 ("Value") 0.0 ("Value")] -> w275
              tunnel: [255.0 ("Value") 1.0 ("Value") 5.0 ("Value")] -> w274
              tunnel: [128.0 ("Value") 0.0 ("Value") 0.0 ("Value")] -> w273
              tunnel: [64.0 ("Value") 0.5 ("Value") 1.0 ("Value")] -> w272
              frame "PWM" {
              }
              frame "Motor", Default {
              }
              frame "Analog Out" {
              }
            }
            n149 = property on="Motor" class="Clust (strict)"("Visible"=TRUE) -> ()  [unwired: 2 in, 2 out]
            n150 = property on="Value" class="Slide (strict)"("Value"=w273, "Scale.Minimum"=w275, "Scale.Maximum"=w274, "Scale.Increment"=w272) -> ()  [unwired: 2 in, 2 out]
            n151 = property on="On/Off" class="Bool (strict)"("Visible"=w277) -> ()  [unwired: 2 in, 2 out]
            n152 = property on="Test Slider" class="Slide (strict)"("Visible"=w277) -> ()  [unwired: 2 in, 2 out]
            n153 = property on="Test Ring" class="Ring (strict)"("Visible"=w277) -> ()  [unwired: 2 in, 2 out]
            n154 = property on="Rev/Fwd" class="Clust (strict)"("Visible"=w277) -> ()  [unwired: 2 in, 2 out]
          }
          frame "Servo" {
            w293 = FALSE ("Visible")
            n155 = call <vilib>:"NT Read Number.vi"("Name"=w295) -> ("Numeric"=w294:dbl)  [unwired: 9 in, 1 out]
            n156 = property on="Test Slider" class="Slide (strict)"("Visible"=TRUE, "Scale.Maximum"=170.0 ("Scale.Range:Maximum")) -> ()  [unwired: 2 in, 2 out]
            n157 = local write "Test Slider"(w294) -> ()
            n158 = property on="Motor" class="Clust (strict)"("Visible"=w293) -> ()  [unwired: 2 in, 2 out]
            n159 = property on="Rev/Fwd" class="Clust (strict)"("Visible"=w293) -> ()  [unwired: 2 in, 2 out]
            n160 = property on="On/Off" class="Bool (strict)"("Visible"=w293) -> ()  [unwired: 2 in, 2 out]
            n161 = property on="Test Ring" class="Ring (strict)"("Visible"=w293) -> ()  [unwired: 2 in, 2 out]
          }
          frame "Relay", "Solenoid" {
            w296 = FALSE ("Visible")
            n162 = property on="Motor" class="Clust (strict)"("Visible"=w296) -> ()  [unwired: 2 in, 2 out]
            n163 = property on="Test Slider" class="Slide (strict)"("Visible"=w296) -> ()  [unwired: 2 in, 2 out]
            n164 = Search and Replace String(input string=w297, search string="/Value  **", replace string="/Direction") -> (result string=w303:string)  [unwired: 5 in, 3 out]
            n165 = property on="Test Ring" class="Ring (strict)"("Visible"=w296) -> ()  [unwired: 2 in, 2 out]
            n166 = call <vilib>:"NT Read String.vi"("Name"=w303) -> ("String"=w301:string)  [unwired: 9 in, 1 out]
            n167 = Equal?(x="Both directions", y=w301) -> (x = y?=w299:bool)
            n168 = Not(x=w299) -> (.not. x?=w300:bool)
            n169 = property on="Rev/Fwd" class="Clust (strict)"("Visible"=w299) -> ()  [unwired: 2 in, 2 out]
            n170 = property on="On/Off" class="Bool (strict)"("Visible"=w300, "Caption.Text"=w298) -> ()  [unwired: 2 in, 2 out]
          }
          frame "Compressor", "Digital Out" {
            w306 = FALSE ("Visible")
            # "Get direction and finish"
            n171 = property on="Motor" class="Clust (strict)"("Visible"=w306) -> ()  [unwired: 2 in, 2 out]
            n172 = property on="Test Slider" class="Slide (strict)"("Visible"=w306) -> ()  [unwired: 2 in, 2 out]
            n173 = property on="Test Ring" class="Ring (strict)"("Visible"=w306) -> ()  [unwired: 2 in, 2 out]
            n174 = property on="On/Off" class="Bool (strict)"("Visible"=TRUE, "Caption.Text"=w307) -> ()  [unwired: 2 in, 2 out]
            n175 = property on="Rev/Fwd" class="Clust (strict)"("Visible"=FALSE) -> ()  [unwired: 2 in, 2 out]
          }
          frame "Camera" {
            n176 = call <vilib>:"Get Last Path Segment.vi"("String in"=w314) -> ("String out"=w315:string)  [unwired: 10 in]
            n177 = property on="On/Off" class="Bool (strict)"("Visible"=FALSE) -> ()  [unwired: 2 in, 2 out]
            n178 = property on="Motor" class="Clust (strict)"("Visible"=FALSE) -> ()  [unwired: 2 in, 2 out]
            n179 = property on="Rev/Fwd" class="Clust (strict)"("Visible"=FALSE) -> ()  [unwired: 2 in, 2 out]
            n180 = case shown="\"White Balance  **\"" w315 {
              tunnel: w314 -> [w321 w330 w339 w348 w357 _ w363]
              tunnel: w313 -> [w319 w327 w336 w345 w354 _ _]
              frame "Size  **" {
                n181 = Index Array(array=w319) -> (element=w318:cluster{string[]})  [unwired: 1 in]
                n182 = call <vilib>:"NT Read String.vi"("Name"=w321) -> ("String"=w320:string)  [unwired: 9 in, 1 out]
                n183 = Unbundle(w318) -> (w316:string[])
                n184 = Match First String(2:w316, 3:w320) -> (0:w317:i32)  [unwired: 1 out]
                n185 = property on="Test Ring" class="Ring (strict)"("Value"=w317, "Strings []"=w316) -> ()  [unwired: 2 in, 2 out]
                n186 = property on="Test Ring" class="Ring (strict)"("Visible"=TRUE) -> ()  [unwired: 2 in, 2 out]
                n187 = property on="Test Slider" class="Slide (strict)"("Visible"=FALSE) -> ()  [unwired: 2 in, 2 out]
              }
              frame "White Balance  **" {
                n188 = Index Array(array=w327, index=1) -> (element=w328:cluster{string[]})
                n189 = call <vilib>:"NT Read String.vi"("Name"=w330) -> ("String"=w329:string)  [unwired: 9 in, 1 out]
                n190 = Unbundle(w328) -> (w325:string[])
                n191 = Match First String(2:w325, 3:w329) -> (0:w324:i32)  [unwired: 1 out]
                n192 = property on="Test Ring" class="Ring (strict)"("Value"=w324, "Strings []"=w325) -> ()  [unwired: 2 in, 2 out]
                n193 = property on="Test Ring" class="Ring (strict)"("Visible"=TRUE) -> ()  [unwired: 2 in, 2 out]
                n194 = property on="Test Slider" class="Slide (strict)"("Visible"=FALSE) -> ()  [unwired: 2 in, 2 out]
              }
              frame "Exposure  **" {
                n195 = Index Array(array=w336, index=2) -> (element=w337:cluster{string[]})
                n196 = call <vilib>:"NT Read String.vi"("Name"=w339) -> ("String"=w338:string)  [unwired: 9 in, 1 out]
                n197 = Unbundle(w337) -> (w333:string[])
                n198 = Match First String(2:w333, 3:w338) -> (0:w334:i32)  [unwired: 1 out]
                n199 = property on="Test Ring" class="Ring (strict)"("Value"=w334, "Strings []"=w333) -> ()  [unwired: 2 in, 2 out]
                n200 = property on="Test Ring" class="Ring (strict)"("Visible"=TRUE) -> ()  [unwired: 2 in, 2 out]
                n201 = property on="Test Slider" class="Slide (strict)"("Visible"=FALSE) -> ()  [unwired: 2 in, 2 out]
              }
              frame "Exposure Priority  **" {
                n202 = Index Array(array=w345, index=3) -> (element=w346:cluster{string[]})
                n203 = call <vilib>:"NT Read String.vi"("Name"=w348) -> ("String"=w347:string)  [unwired: 9 in, 1 out]
                n204 = Unbundle(w346) -> (w342:string[])
                n205 = Match First String(2:w342, 3:w347) -> (0:w343:i32)  [unwired: 1 out]
                n206 = property on="Test Ring" class="Ring (strict)"("Value"=w343, "Strings []"=w342) -> ()  [unwired: 2 in, 2 out]
                n207 = property on="Test Ring" class="Ring (strict)"("Visible"=TRUE) -> ()  [unwired: 2 in, 2 out]
                n208 = property on="Test Slider" class="Slide (strict)"("Visible"=FALSE) -> ()  [unwired: 2 in, 2 out]
              }
              frame "Color Enable  **" {
                n209 = Index Array(array=w354, index=4) -> (element=w355:cluster{string[]})
                n210 = call <vilib>:"NT Read String.vi"("Name"=w357) -> ("String"=w356:string)  [unwired: 9 in, 1 out]
                n211 = Unbundle(w355) -> (w351:string[])
                n212 = Match First String(2:w351, 3:w356) -> (0:w352:i32)  [unwired: 1 out]
                n213 = property on="Test Ring" class="Ring (strict)"("Value"=w352, "Strings []"=w351) -> ()  [unwired: 2 in, 2 out]
                n214 = property on="Test Ring" class="Ring (strict)"("Visible"=TRUE) -> ()  [unwired: 2 in, 2 out]
                n215 = property on="Test Slider" class="Slide (strict)"("Visible"=FALSE) -> ()  [unwired: 2 in, 2 out]
              }
              frame Default {
                n216 = property on="Test Ring" class="Ring (strict)"("Visible"=FALSE) -> ()  [unwired: 2 in, 2 out]
                n217 = property on="Test Slider" class="Slide (strict)"("Visible"=FALSE) -> ()  [unwired: 2 in, 2 out]
              }
              frame "Brightness  **", "Color Level  **", "Compression  **", "FPS  **", "Sharpness  **" {
                n218 = call <vilib>:"NT Read Number.vi"("Name"=w363) -> ("Numeric"=w362:dbl)  [unwired: 9 in, 1 out]
                n219 = local write "Test Slider"(w362) -> ()
                n220 = property on="Test Slider" class="Slide (strict)"("Visible"=TRUE, "Scale.Maximum"=100.0 ("Scale.Range:Maximum")) -> ()  [unwired: 2 in, 2 out]
                n221 = property on="Test Ring" class="Ring (strict)"("Visible"=FALSE) -> ()  [unwired: 2 in, 2 out]
              }
            }
          }
        }
        n222 = property on="Progress" class="Clust (strict)"("Visible"=FALSE) -> ()  [unwired: 2 in, 2 out]
      }
      event "Test Name": Mouse Enter {
        # "Populate the ring with the list of tests"
        n223 = event-data() -> ()  [unwired: 1 in, 1 out]
        n224 = call <vilib>:"NT Read String Array.vi"("Name"="TestMode/TestList") -> ("String Array"=w371:string[])  [unwired: 9 in, 1 out]
        n225 = Build Array (concatenate)("Select the test to run...", w371) -> (w370:string[])
        n226 = property on="Test Name" class="Ring (strict)"("Strings []"=w370) -> ()  [unwired: 2 in, 2 out]
      }
      event "Test Name": Value Change {
        w373 = FALSE ("Visible")
        # "Tell the robot the test name to run"
        n227 = event-data() -> ("NewVal"=w377:u16)  [unwired: 1 in]
        n228 = property on="Test Name" class="Ring (strict)"() -> ("Strings []"=w378:string[])  [unwired: 2 in, 2 out]
        n229 = local write "Progress"(T9 {"Test Progress"=0, "Test Progress Text"=""} ("Progress")) -> ()
        n230 = Index Array(array=w378, index=w377) -> (element=w376:string)
        n231 = call <vilib>:"NT Write String.vi"("String"=w376, "Name"="TestMode/TestName") -> ()  [unwired: 9 in, 1 out]
        n232 = property on="Progress" class="Clust (strict)"("Visible"=TRUE) -> ()  [unwired: 2 in, 2 out]
        n233 = property on="Motor" class="Clust (strict)"("Visible"=w373) -> ()  [unwired: 2 in, 2 out]
        n234 = property on="Test Slider" class="Slide (strict)"("Visible"=w373) -> ()  [unwired: 2 in, 2 out]
        n235 = property on="On/Off" class="Bool (strict)"("Visible"=w373) -> ()  [unwired: 2 in, 2 out]
        n236 = property on="Rev/Fwd" class="Clust (strict)"("Visible"=w373) -> ()  [unwired: 2 in, 2 out]
        n237 = property on="Test Ring" class="Ring (strict)"("Visible"=w373) -> ()  [unwired: 2 in, 2 out]
      }
      event "Start Positions": Mouse Enter {
        # "#competition i broke the wire"
        # "Populate the combo box with the list of autonomous options"
        n238 = event-data() -> ()  [unwired: 1 in, 1 out]
        n239 = disable-structure shown="Disabled" {
          frame Disabled {
            n240 = call <vilib>:"NT Read String Array.vi"("Name"="Auto List") -> ("String Array"=w381:string[])  [unwired: 9 in, 1 out]
            n241 = property on="Start Positions" class="CmbBox"("Strings[]"=w381) -> ()  [unwired: 2 in, 2 out]
          }
          frame Enabled {
          }
        }
      }
      event "Start Positions": Value Change {
        # "User modified the Auto Selection. Write to NT variable so robot knows."
        n242 = event-data() -> ("NewVal"=w383:string)  [unwired: 1 in]
        n243 = call <vilib>:"NT Write String.vi"("String"=w383, "Name"="Auto Selector") -> ()  [unwired: 9 in, 1 out]
      }
      event "Command Selection": Value Change {
        # "Get the params and show in table"
        n244 = event-data() -> ("NewVal"=w389:i32)  [unwired: 1 in]
        n245 = property on="Command Selection" class="MCListbox (strict)"() -> ("ItemNames"=w387:string[][])  [unwired: 2 in, 2 out]
        n246 = call <vilib>:"WPI_DashboardUpdate Command Params.vi"("NewVal"=w389, "Commands"=w387, "Param Tbl"=w388) -> ()  [unwired: 8 in, 1 out]
      }
      event "Execute Command": Value Change {
        # "Started one, Unique ID holds\nresponse"
        n247 = event-data() -> ()  [unwired: 1 in, 1 out]
        n248 = property on="Command Selection" class="MCListbox (strict)"() -> ("ItemNames"=w400:string[][])  [unwired: 2 in, 2 out]
        n249 = Index Array(array=w400, index (row)="Command Selection", index (col)=0) -> (element=w398:string)
        n250 = call <vilib>:"Invoke Commands.vi"("Command Params"="Command Params", "Function Name"=w398) -> ("Params"=w394:u8, "Started"=w393:bool)  [unwired: 7 in, 1 out]
        n251 = Array Subset(array="Command Params", length (row)=w394) -> (w395:string[][])  [unwired: 3 in]
        n252 = Select(t="Executing" ("Cmd Status"), s=w393, f="" ("Cmd Status")) -> (s? t:f=→"Cmd Status":string)
      }
      event "Command Selection": Double Click {
        n253 = event-data() -> ("Row"=w408:i32)  [unwired: 1 in]
        n254 = property on="Command Selection" class="MCListbox (strict)"() -> ("ItemNames"=w411:string[][])  [unwired: 2 in, 2 out]
        n255 = local read "Command Params"() -> (w407:string[][])
        n256 = Index Array(array=w411, index (row)=w408, index (col)=0) -> (element=w409:string)
        n257 = call <vilib>:"Invoke Commands.vi"("Command Params"=w407, "Function Name"=w409) -> ("Params"=w406:u8, "Started"=w401:bool)  [unwired: 7 in, 1 out]
        n258 = Array Subset(array=w407, length (row)=w406) -> (w405:string[][])  [unwired: 3 in]
        n259 = Select(t="Executing" ("Cmd Status"), s=w401, f="" ("Cmd Status")) -> (s? t:f=w402:string)
        n260 = local write "Cmd Status"(w402) -> ()
      }
      event "CheckList": Double Click {
        # "Shift clears all"
        # "Update symbols on the listbox"
        n261 = event-data() -> ("PlatMods.Shift"=w413:bool, "Row"=w415:i32)  [unwired: 1 in]
        n262 = case shown="True" w413 {
          tunnel: w415 -> [w419 _]
          tunnel: 1 -> [w418 _]
          frame False {
            n263 = property on="CheckList" class="LstBox (strict)"() -> ("Item Symbols"=w417:i32[])  [unwired: 2 in, 2 out]
            n264 = Replace Array Subset(array=w417, new element=w418, index=w419) -> (w416:i32[])
            n265 = property on="CheckList" class="LstBox (strict)"("Item Symbols"=w416) -> ()  [unwired: 2 in, 2 out]
          }
          frame True {
            w420 = 0 ("Top Row")
            n266 = property on="CheckList" class="LstBox (strict)"() -> ("Number of Rows"=w422:u32)  [unwired: 2 in, 2 out]
            n267 = Initialize Array(0, w422) -> (w421:i32[])
            n268 = property on="CheckList" class="LstBox (strict)"("Top Row"=w420, "Value"=w420, "Item Symbols"=w421) -> ()  [unwired: 2 in, 2 out]
          }
        }
      }
      event "CheckList": Key Down {
        # "Update symbols on the listbox\nLeft and right keys check and uncheck"
        n269 = event-data() -> ("VKey"=w426:T25)  [unwired: 1 in]
        n270 = case shown="\"Left\", \"Right\"" w426 {
          selector: w426 -> [w431 _]
          tunnel: eventvkey."Left" ("VKey") -> [w429 _]
          frame "Left", "Right" {
            n271 = Equal?(x=w429, y=w431) -> (x = y?=w430:bool)
            n272 = Select(t=0, s=w430, f=1) -> (s? t:f=w432:i32)
            n273 = property on="CheckList" class="LstBox (strict)"() -> ("Item Symbols"=w435:i32[])  [unwired: 2 in, 2 out]
            n274 = Replace Array Subset(array=w435, new element=w432, index="CheckList") -> (w434:i32[])
            n275 = property on="CheckList" class="LstBox (strict)"("Item Symbols"=w434) -> ()  [unwired: 2 in, 2 out]
          }
          frame Default {
          }
        }
      }
      event "Motor.Enable": Value Change {
        # "When the test mode otor enable helper is set, update that\ntree row item's value"
        n276 = event-data() -> ("NewVal"=w441:bool)  [unwired: 1 in]
        n277 = Unbundle("Motor") -> ("Value"=w440:dbl)  [unwired: 1 out]
        n278 = Select(t=w440, s=w441, f=0.0) -> (s? t:f=w438:dbl)
        n279 = call <vilib>:"NT Write Number.vi"("Numeric"=w438, "Name"=w437) -> ()  [unwired: 9 in, 1 out]
      }
      event "Test Slider": Value Change {
        # "When the test mode slider helper is set, update that\ntree row item's value"
        n280 = event-data() -> ("NewVal"=w444:dbl)  [unwired: 1 in]
        n281 = call <vilib>:"NT Write Number.vi"("Numeric"=w444, "Name"=w445) -> ()  [unwired: 9 in, 1 out]
      }
      event "On/Off": Value Change {
        # "When the test mode on/off helper value is set, update that\ntree row item's value"
        n282 = event-data() -> ("NewVal"=w449:bool)  [unwired: 1 in]
        n283 = Boolean To (0,1)(Boolean=w449) -> (0, 1=w448:i16)
        n284 = call <vilib>:"NT Write Number.vi"("Numeric"=w448, "Name"=w447) -> ()  [unwired: 9 in, 1 out]
      }
      event "Rev/Fwd": Value Change {
        # "When the test mode helper value for relays is set, update that\ntree row item's value"
        n285 = event-data() -> ("NewVal.Forward"=w457:bool, "NewVal.Reverse"=w456:bool)  [unwired: 1 in]
        n286 = Boolean To (0,1)(Boolean=w457) -> (0, 1=w453:i16)
        n287 = Boolean To (0,1)(Boolean=w456) -> (0, 1=w455:i16)
        n288 = Negate(x=w455) -> (-x=w454:i16)
        n289 = Add(x=w453, y=w454) -> (x+y=w452:i16)
        n290 = call <vilib>:"NT Write Number.vi"("Numeric"=w452, "Name"=w451) -> ()  [unwired: 9 in, 1 out]
      }
      event "Test Ring": Value Change {
        # "When a test mode helper value is selected from the ring,\nset the tree item's variable to the string value"
        n291 = event-data() -> ("NewVal"=w461:u16)  [unwired: 1 in]
        n292 = property on="Test Ring" class="Ring (strict)"() -> ("Strings []"=w462:string[])  [unwired: 2 in, 2 out]
        n293 = Index Array(array=w462, index=w461) -> (element=w460:string)
        n294 = call <vilib>:"NT Write String.vi"("String"=w460, "Name"=w459) -> ()  [unwired: 9 in, 1 out]
      }
      event "Rec Mode": Value Change {
        # "Update globals for recording mode and path to read log from.\nClear when logging and let NetworkTables set path for vision to\nuse."
        n295 = event-data() -> ("NewVal"=w473:enum32{"Stop", "Record", "Playback"})  [unwired: 1 in]
        n296 = global write "WPI_DashboardLogging Global.vi" "Logging Filename"(path "") -> ()
        n297 = global write "WPI_DashboardLogging Global.vi" "Recording"(w473) -> ()
        n298 = case shown="\"Playback\"" w473 {
          tunnel: w472 -> [_ w475 w484]
          tunnel: [_ _ w483] -> w470
          tunnel: [_ _ w482] -> _
          tunnel: w468 -> [_ _ w480]
          tunnel: cluster{i32, i32} {-250, 170} -> [_ _ w479]
          tunnel: [_ _ T26 {"Image Size"=TRUE, "Image Type"=TRUE, "Pixel Value"=TRUE, "ROI Information"=TRUE, "Zoom Factor"=FALSE} ("Image Information Shown:All Elements")] -> w463
          tunnel: [_ _ TRUE ("Zoom Factor")] -> w464
          tunnel: w466 -> [_ _ w476]
          frame Default {
          }
          frame "Stop", "Record" {
            # "Place Window too"
            n299 = invoke class="VI" method="FP.Close"(reference=w475) -> (reference out=w474:refnum<vi>)  [unwired: 2 in, 2 out]
            n300 = invoke class="VI" method="Abort VI"(reference=w474) -> ()  [unwired: 2 in, 3 out]
          }
          frame "Playback" {
            n301 = call "Open Playback Panel.vi"("Offset"=w479, "DB VI Ref"=w480, "Playback in"=w484) -> ("Playback out"=w481:refnum<vi>)  [unwired: 8 in]
            n302 = register-events(w481, w476) -> (reference out=w483:refnum<event-registration>, error out=w482:errorcluster)  [unwired: 2 in]
          }
        }
        n303 = property on="Camera Image Right" class="ImageControl"("Image Information Shown"=w463, "Image Information Visible"=w464) -> ()  [unwired: 2 in, 2 out]
        n304 = property on="Camera Image" class="ImageControl"("Image Information Shown"=w463, "Image Information Visible"=w464) -> ()  [unwired: 2 in, 2 out]
        n305 = call <vilib>:"WPI_DashboardNT Log FieldName Cache.vi"("Operation"=enum16{"Lookup/Add", "Index", "Clear"}."Clear") -> ()  [unwired: 8 in, 3 out]
      }
      event Panel Close {
        w486 = enum32{"Stop", "Record", "Playback"}."Stop" ("Rec Mode")
        # "Playback window has been closed, abort"
        n306 = event-data() -> ()  [unwired: 1 in, 4 out]
        n307 = local write "Rec Mode"(w486) -> ()
        n308 = global write "WPI_DashboardLogging Global.vi" "Recording"(w486) -> ()
      }
      event Panel Close {
        # "Abort playback window and ourself"
        n309 = event-data() -> ()  [unwired: 1 in, 4 out]
        n310 = invoke class="VI" method="FP.Close"(reference=w490) -> (reference out=w489:refnum<vi>)  [unwired: 2 in, 2 out]
        n311 = invoke class="VI" method="Abort VI"(reference=w489) -> (error out=w488:errorcluster)  [unwired: 2 in, 2 out]
        n312 = invoke class="VI" method="Abort VI"(error in=w488) -> ()  [unwired: 2 in, 3 out]
      }
      event User Event {
        n313 = event-data() -> ("IDs"=w497:cluster{"RPC field ID":u16, "Unique ID":u16}, "String"=w496:string)  [unwired: 1 in]
        n314 = Bundle("IDs"=w497, "String"=w496) -> (w495:T13)  [unwired: 1 in]
        n315 = call <vilib>:"Retrieve RPC Response.vi"("RPC Response"=w495) -> ("Output"=w493:string[][])  [unwired: 10 in]
        n316 = Build Array (concatenate)(w491, w493) -> (w492:string[][])
        n317 = local write "Command Params"(w492) -> ()
        n318 = local write "Cmd Status"("" ("Cmd Status")) -> ()
      }
      event "Tree": Double Click {
        n319 = event-data() -> ("PlatMods"=w503:T29, "Tag"=w500:string)  [unwired: 1 in]
        n320 = Unbundle(w503) -> ("Shift"=w502:bool)  [unwired: 4 out]
        n321 = String Subset(string=w500, length (rest)=1 ("length (rest)")) -> (substring=w499:string)  [unwired: 1 in]
        n322 = Not(x=w502) -> (.not. x?=w501:bool)
        n323 = case shown="\"/\"" w499 {
          tunnel: w500 -> [_ w506]
          tunnel: w501 -> [_ w505]
          frame Default {
          }
          frame "/" {
            n324 = call <vilib>:"NT Update Persistence.vi"("Persistence"=w505, "Name"=w506) -> ()  [unwired: 9 in, 1 out]
          }
        }
      }
    }
  }
  n325 = while {
    tunnel: w65 -> [w508]
    i -> [w511]
    stop <- FALSE stop-if-true
    n326 = Wait (ms)(milliseconds to wait=u32 100) -> ()  [unwired: 1 out]
    n327 = case shown="\"Playback\"" "Rec Mode" {
      tunnel: w511 -> [_ _ w526]
      tunnel: [u32 2829099 ("Base Color") u32 11141120 ("Target Color") w515] -> w507
      frame "Stop", Default {
        # "Reset the color, extra updates don't cost much"
      }
      frame "Record" {
      }
      frame "Playback" {
        # "Playback"
        n328 = Quotient & Remainder(x=w526, y=u32 50 ("milliseconds to wait")) -> (x-y*floor(x/y)=w522:u32)  [unwired: 1 out]
        n329 = Divide(x=w522, y=u32 50 ("milliseconds to wait")) -> (x/y=w519:dbl)
        n330 = Multiply(x=6.283185307179586, y=w519) -> (x*y=w524:dbl)
        n331 = Sine(x=w524) -> (sin(x)=w523:dbl)
        n332 = Absolute Value(x=w523) -> (abs(x)=w516:dbl)
        n333 = call "Interpolate RGB Color.vi"("Proportion"=w516, "Target Color"=u32 30976, "Base Color"=u32 2829099) -> ("Result Color"=w515:u32)  [unwired: 8 in]
      }
    }
    n334 = property class="Pane"(reference=w508, "PaneColor"=w507) -> ()  [unwired: 1 in, 2 out]
  }
  n335 = local write "Dashboard Tab"(T2."Drive" ("Dashboard Tab")) -> ()
  n336 = property on="On/Off" class="Bool (strict)"("Visible"=w38) -> ()  [unwired: 2 in, 2 out]
  n337 = property on="Motor" class="Clust (strict)"("Visible"=w38) -> ()  [unwired: 2 in, 2 out]
  n338 = property on="Progress" class="Clust (strict)"("Visible"=w38) -> ()  [unwired: 2 in, 2 out]
  n339 = property on="Test Ring" class="Ring (strict)"("Visible"=w38) -> ()  [unwired: 2 in, 2 out]
  n340 = property on="Rev/Fwd" class="Clust (strict)"("Visible"=w38) -> ()  [unwired: 2 in, 2 out]
  n341 = local write "Command Selection"(u16 0 ("milliseconds to wait")) -> ()
  n342 = while {
    tunnel: u16 1741 ("timeout ms (25000)") -> [w528]
    stop <- FALSE stop-if-true
    n343 = TCP Create Listener(10:w528) -> (0:w527:errorcluster, 3:w529:refnum<k5>)  [unwired: 4 in, 1 out]
    n344 = case shown="No Error" w527 {
      selector: w527 -> [w531 _]
      tunnel: w529 -> [w532 _]
      frame No Error {
        n345 = while {
          tunnel: w532 -> [w535]
          tunnel: w531 -> [w534]
          stop <- FALSE stop-if-true
          n346 = TCP Wait On Listener(8:w534, 11:w535) -> (0:w536:errorcluster, 4:w537:refnum<k5>)  [unwired: 2 in, 3 out]
          n347 = local write "TCP"(w537) -> ()
          n348 = case shown="No Error" w536 {
            frame No Error {
            }
            frame Error {
              n349 = Wait (ms)(milliseconds to wait=u32 1000) -> ()  [unwired: 1 out]
            }
          }
        }
      }
      frame Error {
        n350 = Wait (ms)(milliseconds to wait=u32 1000) -> ()  [unwired: 1 out]
      }
    }
  }
  n351 = local write "Command Params"(string[][] [] ("Command Params")) -> ()
  n352 = global write "WPI_DashboardLogging Global.vi" "Recording"(w59) -> ()
  n353 = local write "Rec Mode"(w59) -> ()
  n354 = while {
    stop <- FALSE stop-if-true
    # "haha do you guys not know what\nabsolute values are?"
    # "squam's code :) (its not bad)"
    # "hello thank you"
    n355 = Absolute Value(x="Auto Wait") -> (abs(x)=w540:dbl)
    n356 = call-poly <vilib>:"NT Write Value.vi"("Numeric"=w540, "Name"="Auto Delay") -> ()  [unwired: 9 in, 1 out]
  }
  n357 = while {
    stop <- FALSE stop-if-true
    n358 = call <vilib>:"NT Write String.vi"("String"="Start Positions", "Name"="Position Selector") -> ()  [unwired: 9 in, 1 out]
  }
  n359 = while {
    stop <- FALSE stop-if-true
    n360 = call <vilib>:"NT Write String.vi"("String"="Auton Goalos", "Name"="Auto Selector") -> ()  [unwired: 9 in, 1 out]
  }
  n361 = call <vilib>:"Get_LinearAcceleration.vi"("Device Number"=FRIC_navX_DeviceNumbersTypeDef."Dev0", "Update"=TRUE) -> ("Linear Acceleration"=→"Linear Acceleration":T5)  [unwired: 9 in]
